vi "Generate Request ID.vi"(8 "error in (no error)":errorcluster) -> (0 "error out":errorcluster, 3 "Request ID":u32)   [LabVIEW 2020, in "Publisher.lvlib" / "Request Reply Core.lvclass"]
doc: "Generate a Request ID as a U32 numeric.\n0 is returned on error."
uses:
  Request Reply Core.lvclass
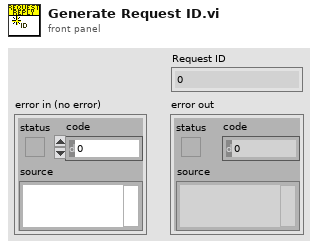
[diagram p1: front panel]
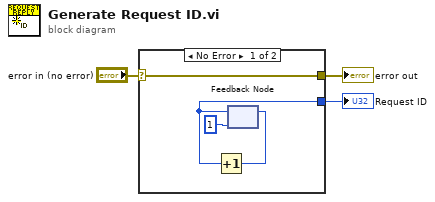
[diagram p0: block diagram]
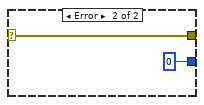
[diagram p2: hidden frame]
diagram:
  n1 = case shown="No Error" "error in (no error)" {
    selector: "error in (no error)" -> [w7 w9]
    tunnel: [w7 w9] -> w2
    tunnel: [w5 u32 0 ("Request ID")] -> w1
    frame No Error {
      n2 = feedback #1(u32 1 ("Request ID")) -> (w5:u32)
      n3 = Increment(x=w5) -> (x+1=w4:u32)
      n4 = feedback-in #1(w4) -> ()
    }
    frame Error {
    }
  }
  "error out" <- w2
  "Request ID" <- w1
